vi "Simple Scripting Example - Add on LabVIEW Side.vi"() -> ()   [LabVIEW 2013]
uses:
  LabVIEW Core/TS.lvlib
  LabVIEW Core/LabVIEW Python Connector Message.ctl
panel:
  out "error out":errorcluster
  out "Sum":string
  # "LabVIEW will add:\n3 + 4 + 5"
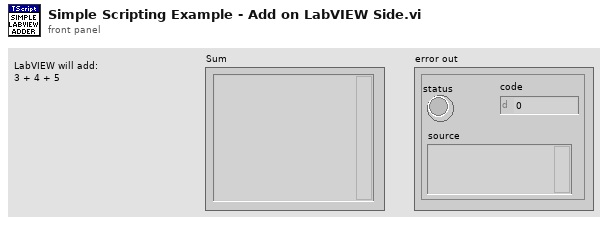
[diagram p1: front panel]
types:
  T1 = typedef "TS.lvlib/LabVIEW Python Connector Message.ctl" = cluster{"Command":string, "Data":string[], "Script ID":i64, "LabVIEW Server ID":string, "Python Message ID":i32}
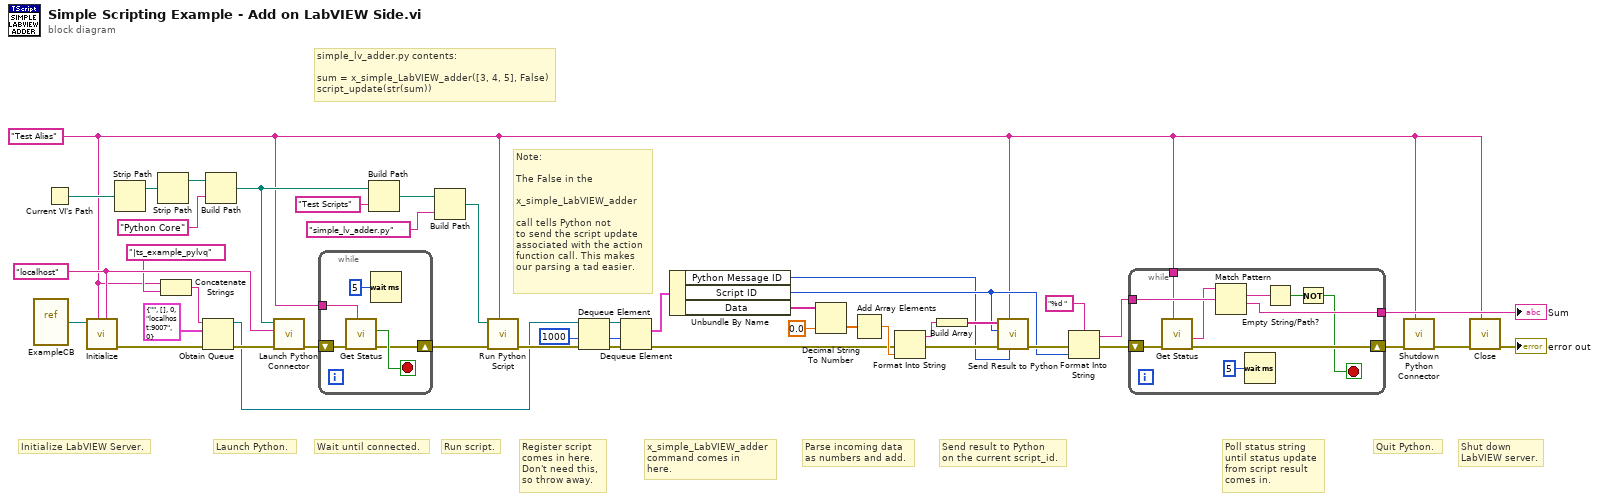
[diagram p0: block diagram]
diagram:
  w1 = "Test Alias"
  w22 = 1000 ("timeout in ms (-1)")
  w36 = "localhost" ("IP Address for LabVIEW Server")
  # "Send result to Python\non the current script_id."
  # "Parse incoming data\nas numbers and add."
  # "x_simple_LabVIEW_adder\ncommand comes in\nhere."
  # "Note: \n\nThe False in the \n\nx_simple_LabVIEW_adder\n\ncall tells Python not\nto send the script update\nassociated with the action\nfunction call. This makes \nour parsing a tad easier."
  # "simple_lv_adder.py contents:\n\nsum = x_simple_LabVIEW_adder([3, 4, 5], False)\nscript_update(str(sum))"
  # "Shut down\nLabVIEW server."
  # "Quit Python."
  # "Poll status string\nuntil status update\nfrom script result\ncomes in."
  # "Register script\ncomes in here.\nDon't need this,\nso throw away."
  # "Run script."
  # "Wait until connected."
  # "Launch Python."
  # "Initialize LabVIEW Server."
  n1 = vi-ref "ExampleCB.vi"() -> (w5:refnum<vi>)
  n2 = Current VI's Path() -> (path=w37:path)
  n3 = call "Initialize.vi"("IP Address for LabVIEW Server"=w36, "Server Alias"=w1, "VI Refnum"=w5) -> ("error out"=w42:errorcluster)  [unwired: 8 in]
  n4 = Strip Path(path=w37) -> (stripped path=w39:path)  [unwired: 1 out]
  n5 = Strip Path(path=w39) -> (stripped path=w40:path)  [unwired: 1 out]
  n6 = Concatenate Strings(w1, "|ts_example_pylvq" ("name (unnamed)")) -> (w2:string)
  n7 = Obtain Queue(name (unnamed)=w2, element data type=T1 {"Command"="", "Data"=[], "Script ID"=0, "LabVIEW Server ID"="localhost:9007", "Python Message ID"=0} ("element"), error in (no error)=w42) -> (queue out=w27:refnum<queue>, error out=w41:errorcluster)  [unwired: 2 in, 1 out]
  n8 = Build Path(base path=w40, name or relative path="Python Core") -> (appended path=w35:path)
  n9 = call "Launch Python Connector.vi"("error in (no error)"=w41, "Tell Python the IP Address Where LabVIEW Is"=w36, "Path to Python Core Folder"=w35) -> ("error out"=w30:errorcluster)  [unwired: 8 in]
  n10 = while {
    shift-right: [w46] -> w29
    shift-left: w30 -> [w48]
    tunnel: w1 -> [w44]
    stop <- w47 stop-if-true
    n11 = call "Get Status.vi"("Server Alias"=w44, "error in (no error)"=w48) -> ("error out"=w46:errorcluster, "Connected"=w47:bool)  [unwired: 4 in, 4 out]
    n12 = Wait (ms)(milliseconds to wait=u32 5) -> ()  [unwired: 1 out]
  }
  n13 = Build Path(base path=w35, name or relative path="Test Scripts") -> (appended path=w33:path)
  n14 = Build Path(base path=w33, name or relative path="simple_lv_adder.py") -> (appended path=w31:path)
  n15 = call "Run Python Script.vi"("Server Alias"=w1, "error in (no error)"=w29, "Absolute Python Script Path"=w31) -> ("error out"=w28:errorcluster)  [unwired: 8 in]
  n16 = Dequeue Element(queue=w27, timeout in ms (-1)=w22, error in (no error)=w28) -> (queue out=w24:refnum<queue>, error out=w23:errorcluster)  [unwired: 2 out]
  n17 = Dequeue Element(queue=w24, timeout in ms (-1)=w22, error in (no error)=w23) -> (element=w21:T1, error out=w14:errorcluster)  [unwired: 2 out]
  n18 = Unbundle By Name(w21) -> ("Python Message ID"=w4:i32, "Script ID"=w10:i64, "Data"=w13:string[])
  n19 = Decimal String To Number(string=w13, default (0L)=0.0) -> (number=w16:dbl[])  [unwired: 1 in, 1 out]
  n20 = Add Array Elements(numeric array=w16) -> (sum=w17:dbl)
  n21 = Format Into String(error in=w14, w17) -> (resulting string=w19:string, error out=w18:errorcluster)  [unwired: 2 in]
  n22 = Build Array(w19) -> (w20:string[])
  n23 = call "Send Result to Python.vi"("Python Message ID"=w4, "Server Alias"=w1, "error in (no error)"=w18, "Script ID"=w10, "Result Data"=w20) -> ("error out"=w11:errorcluster)  [unwired: 6 in]
  n24 = Format Into String(format string="%d ", error in=w11, w10) -> (resulting string=w9:string, error out=w8:errorcluster)  [unwired: 1 in]
  n25 = while {
    shift-right: [w52] -> w6
    shift-left: w8 -> [w58]
    tunnel: w9 -> [w57]
    tunnel: [w54] -> w7
    tunnel: w1 -> [w49]
    stop <- w50 stop-if-true
    n26 = call "Get Status.vi"("Server Alias"=w49, "error in (no error)"=w58) -> ("error out"=w52:errorcluster, "Script Status"=w56:string)  [unwired: 4 in, 4 out]
    n27 = Match Pattern(string=w56, regular expression=w57) -> (match substring=w55:string, after substring=w54:string)  [unwired: 1 in, 2 out]
    n28 = Wait (ms)(milliseconds to wait=u32 5) -> ()  [unwired: 1 out]
    n29 = Empty String/Path?(string/path=w55) -> (empty?=w53:bool)
    n30 = Not(x=w53) -> (.not. x?=w50:bool)
  }
  "Sum" <- w7
  n31 = call "Shutdown Python Connector.vi"("Server Alias"=w1, "error in (no error)"=w6) -> ("error out"=w26:errorcluster)  [unwired: 9 in]
  n32 = call "Close.vi"("Server Alias"=w1, "error in (no error)"=w26) -> ("error out"=→"error out":errorcluster)  [unwired: 9 in]
